vi "Dynamic Load Log Record.vi"(8 "Error In":errorcluster) -> (0 "Error Out":errorcluster, 2 "Device names":string[](array[string]), 3 "Digitizers out":refnum<class "Process Object.lvclass">[](array[class]))   [LabVIEW 2020]
uses:
  Process Object/Process Object.lvclass
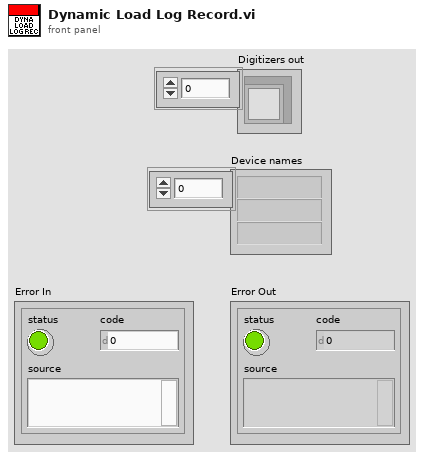
[diagram p1: front panel]
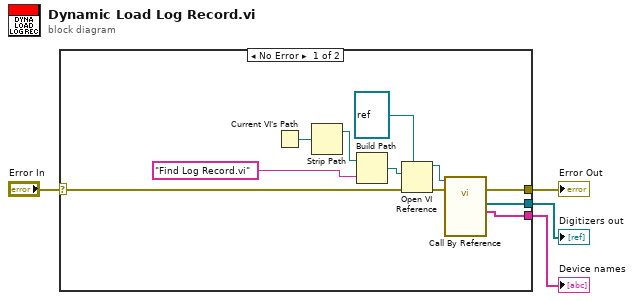
[diagram p0: block diagram]
diagram:
  n1 = case shown="No Error" "Error In" {
    selector: "Error In" -> [w12 w16]
    tunnel: [w15 w16] -> w2
    tunnel: [w14 _] -> w4
    tunnel: [w13 _] -> w3
    frame No Error {
      n2 = Current VI's Path() -> (path=w10:path)
      n3 = Strip Path(path=w10) -> (stripped path=w5:path)  [unwired: 1 out]
      n4 = Build Path(base path=w5, name or relative path="Find Log Record.vi") -> (appended path=w6:path)
      n5 = Open VI Reference(type specifier VI Refnum (for type only)=refnum<vi> refnum, vi path=w6, error in (no error)=w12) -> (vi reference=w8:refnum<vi>, error out=w7:errorcluster)  [unwired: 3 in]
      n6 = call-by-ref "?"(reference=w8, error in=w7) -> (error out=w15:errorcluster, "Names"=w14:string[], "Module List"=w13:refnum<class "Process Object.lvclass">[])  [unwired: 9 in, 2 out]
    }
    frame Error {
    }
  }
  "Error Out" <- w2
  "Digitizers out" <- w3
  "Device names" <- w4
